vi "TestM1M3SALTelemetry.vi"() -> ()   [LabVIEW 2016]
uses:
  Communicator/M1M3SAL/M1M3SAL.lvclass
  Communicator/DataTypes/M1M3SALSettings.ctl
  UserEvents/UserEvents.lvclass
  DataTypes/General/ShutdownEvent.ctl
  Communicator/M1M3SAL/M1M3SAL.lvclass/M1M3SAL.ctl
  UserEvents/UserEvents.lvclass/UserEvents.ctl
  DataTypes/Topics/TelemetryAirData.ctl
  DataTypes/Topics/Parts/Timestamp.ctl
  DataTypes/Topics/TelemetryIMSData.ctl
  DataTypes/Topics/TelemetryDynamicData.ctl
  DataTypes/Topics/TelemetryElevationData.ctl
  DataTypes/Topics/TelemetryForceActuatorData.ctl
  DataTypes/Topics/TelemetryForceActuatorStatus.ctl
  DataTypes/Topics/TelemetryFPGAData.ctl
  DataTypes/Topics/TelemetryMirrorForceData.ctl
  DataTypes/Topics/TelemetryHardpointData.ctl
  DataTypes/Topics/TelemetryHardpointStatus.ctl
  Communicator/M1M3SupportCommunicator.lvlib
  DataTypes/Topics/M1M3SupportTopics.lvlib
  DataTypes/General/M1M3SupportGeneral.lvlib
panel:
  out "TelemetryMirrorForceData":bool
  in  "TelemetryMirrorForceDataGo":bool
  out "TelemetryHardpointStatus":bool
  out "TelemetryHardpointData":bool
  out "TelemetryFPGAData":bool
  in  "TelemetryHardpointStatus":bool
  in  "TelemetryHardpointData":bool
  in  "TelemetryFPGADataGo":bool
  out "TelemetryForceActuatorStatus":bool
  out "TelemetryForceActuatorData":bool
  out "TelemetryElevationData":bool
  out "TelemetryDynamicData":bool
  in  "TelemetryForceActuatorStatusGo":bool
  in  "TelemetryForceActuatorDataGo":bool
  in  "TelemetryElevationDataGo":bool
  in  "TelemetryDynamicDataGo":bool
  in  "TelemetryIMSDataGo":bool
  out "TelemetryIMSData":bool
  out "Ready?":bool
  in  "TelemetryAirDataGo":bool
  out "TelemetryAirData":bool
  in  "Stop":bool
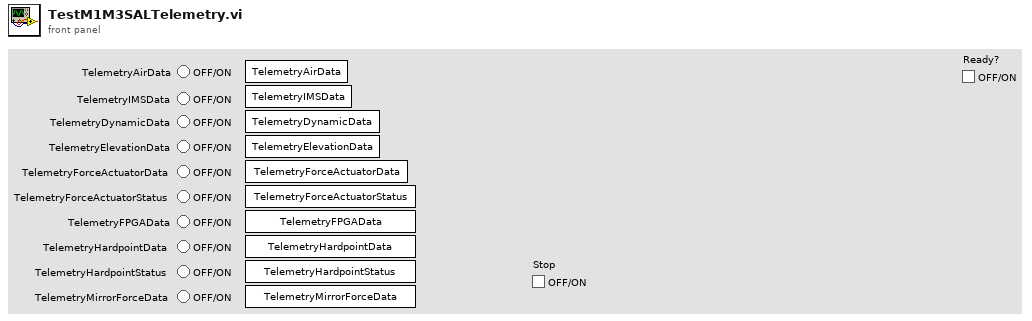
[diagram p1: front panel]
types:
  T1 = typedef "M1M3SupportGeneral.lvlib/ShutdownEvent.ctl" = cluster{"Shutdown":bool}
  T2 = typedef "M1M3SupportCommunicator.lvlib/M1M3SALSettings.ctl" = cluster{"IPAddress":string, "Port":u16, "StartupScript":string}
  T3 = typedef "M1M3SupportTopics.lvlib/Timestamp.ctl" = dbl
  T4 = typedef "M1M3SupportTypes.lvlib/Timestamp.ctl" = dbl
  T5 = typedef "M1M3SupportTopics.lvlib/TelemetryAirData.ctl" = cluster{"Timestamp":T3, "CellAirPressure":sgl, "HardpointAirPressure":sgl}
  T6 = typedef "M1M3SupportTopics.lvlib/TelemetryIMSData.ctl" = cluster{"Timestamp":T3, "XPosition":dbl, "YPosition":dbl, "ZPosition":dbl, "XRotation":dbl, "YRotation":dbl, "ZRotation":dbl}
  T7 = typedef "M1M3SupportTopics.lvlib/TelemetryDynamicData.ctl" = cluster{"Timestamp":T3, "AzimuthVelocity":dbl, "ElevationVelocity":dbl, "AzimuthAcceleration":dbl, "ElevationAcceleration":dbl}
  T8 = typedef "M1M3SupportTopics.lvlib/TelemetryElevationData.ctl" = cluster{"Timestamp":T3, "InclinometerElevation":dbl, "MeasuredElevation":dbl}
  T9 = typedef "M1M3SupportTopics.lvlib/TelemetryForceActuatorData.ctl" = cluster{"Timestamp":T3, "SlewFlagCommanded":bool[], "XSetpointCommanded":dbl[], "YSetpointCommanded":dbl[], "ZSetpointCommanded":dbl[], "XForce":sgl[], "YForce":sgl[], "ZForce":sgl[], "ILCFault":bool[], "DCAFault":bool[], "BroadcastCounter":u8[]}
  T10 = typedef "M1M3SupportTopics.lvlib/TelemetryForceActuatorStatus.ctl" = cluster{"Timestamp":T3, "Mode":u8[], "MajorFault":bool[], "MinorFault":bool[], "FaultOverridden":bool[], "DCAFault":bool[], "WatchdogReset":bool[], "BrownoutDetected":bool[], "EventTrapReset":bool[], "MotorPowerFault":bool[], "SSRPowerFault":bool[], "AUXPowerFault":bool[], "SMCPowerFault":bool[], "DCAOutputsEnabled":bool[], "DCAPowerFault":bool[], "DCAAmplifierAFault":bool[], "DCAAmplifierBFault":bool[], "DCAEventTrapReset":bool[]}
  T11 = typedef "M1M3SupportTopics.lvlib/TelemetryFPGAData.ctl" = cluster{"Timestamp":T3, "ModbusSubnetATxInternalFIFOOverflow":bool, "ModbusSubnetAInvalidInstruction":bool, "ModbusSubnetAWaitForRxFrameTimeout":bool, "ModbusSubnetAStartBitError":bool, "ModbusSubnetAStopBitError":bool, "ModbusSubnetARxDataFIFOOverflow":bool, "ModbusSubnetATxByteCount":u32, "ModbusSubnetATxFrameCount":u32, "ModbusSubnetARxByteCount":u32, "ModbusSubnetARxFrameCount":u32, "ModbusSubnetBTxInternalFIFOOverflow":bool, "ModbusSubnetBInvalidInstruction":bool, "ModbusSubnetBWaitForRxFrameTimeout":bool, "ModbusSubnetBStartBitError":bool, "ModbusSubnetBStopBitError":bool, "ModbusSubnetBRxDataFIFOOverflow":bool, "ModbusSubnetBTxByteCount":u32, "ModbusSubnetBTxFrameCount":u32, "ModbusSubnetBRxByteCount":u32, "ModbusSubnetBRxFrameCount":u32, "ModbusSubnetCTxInternalFIFOOverflow":bool, "ModbusSubnetCInvalidInstruction":bool, "ModbusSubnetCWaitForRxFrameTimeout":bool, "ModbusSubnetCStartBitError":bool, "ModbusSubnetCStopBitError":bool, "ModbusSubnetCRxDataFIFOOverflow":bool, "ModbusSubnetCTxByteCount":u32, "ModbusSubnetCTxFrameCount":u32, "ModbusSubnetCRxByteCount":u32, "ModbusSubnetCRxFrameCount":u32, "ModbusSubnetDTxInternalFIFOOverflow":bool, "ModbusSubnetDInvalidInstruction":bool, "ModbusSubnetDWaitForRxFrameTimeout":bool, "ModbusSubnetDStartBitError":bool, "ModbusSubnetDStopBitError":bool, "ModbusSubnetDRxDataFIFOOverflow":bool, "ModbusSubnetDTxByteCount":u32, "ModbusSubnetDTxFrameCount":u32, "ModbusSubnetDRxByteCount":u32, "ModbusSubnetDRxFrameCount":u32, "ModbusSubnetETxInternalFIFOOverflow":bool, "ModbusSubnetEInvalidInstruction":bool, "ModbusSubnetEWaitForRxFrameTimeout":bool, "ModbusSubnetEStartBitError":bool, "ModbusSubnetEStopBitError":bool, "ModbusSubnetERxDataFIFOOverflow":bool, "ModbusSubnetETxByteCount":u32, "ModbusSubnetETxFrameCount":u32, "ModbusSubnetERxByteCount":u32, "ModbusSubnetERxFrameCount":u32, "FPGATimestamp":dbl}
  T12 = typedef "M1M3SupportTopics.lvlib/TelemetryMirrorForceData.ctl" = cluster{"Timestamp":T3, "Fx":dbl, "Fy":dbl, "Fz":dbl, "Mx":dbl, "My":dbl, "Mz":dbl}
  T13 = typedef "M1M3SupportTopics.lvlib/TelemetryHardpointData.ctl" = cluster{"Timestamp":T3, "StepsCommanded":i16[], "Force":sgl[], "Encoder":i32[], "ILCFault":bool[], "CWLimitOperated":bool[], "CCWLimitOperated":bool[], "BroadcastCounter":u8[]}
  T14 = typedef "M1M3SupportTopics.lvlib/TelemetryHardpointStatus.ctl" = cluster{"Timestamp":T3, "Mode":u8[], "MajorFault":bool[], "MinorFault":bool[], "FaultOverridden":bool[], "WatchdogReset":bool[], "BrownoutDetected":bool[], "EventTrapReset":bool[], "MotorPowerFault":bool[], "SSRPowerFault":bool[], "AUXPowerFault":bool[], "SMCPowerFault":bool[]}
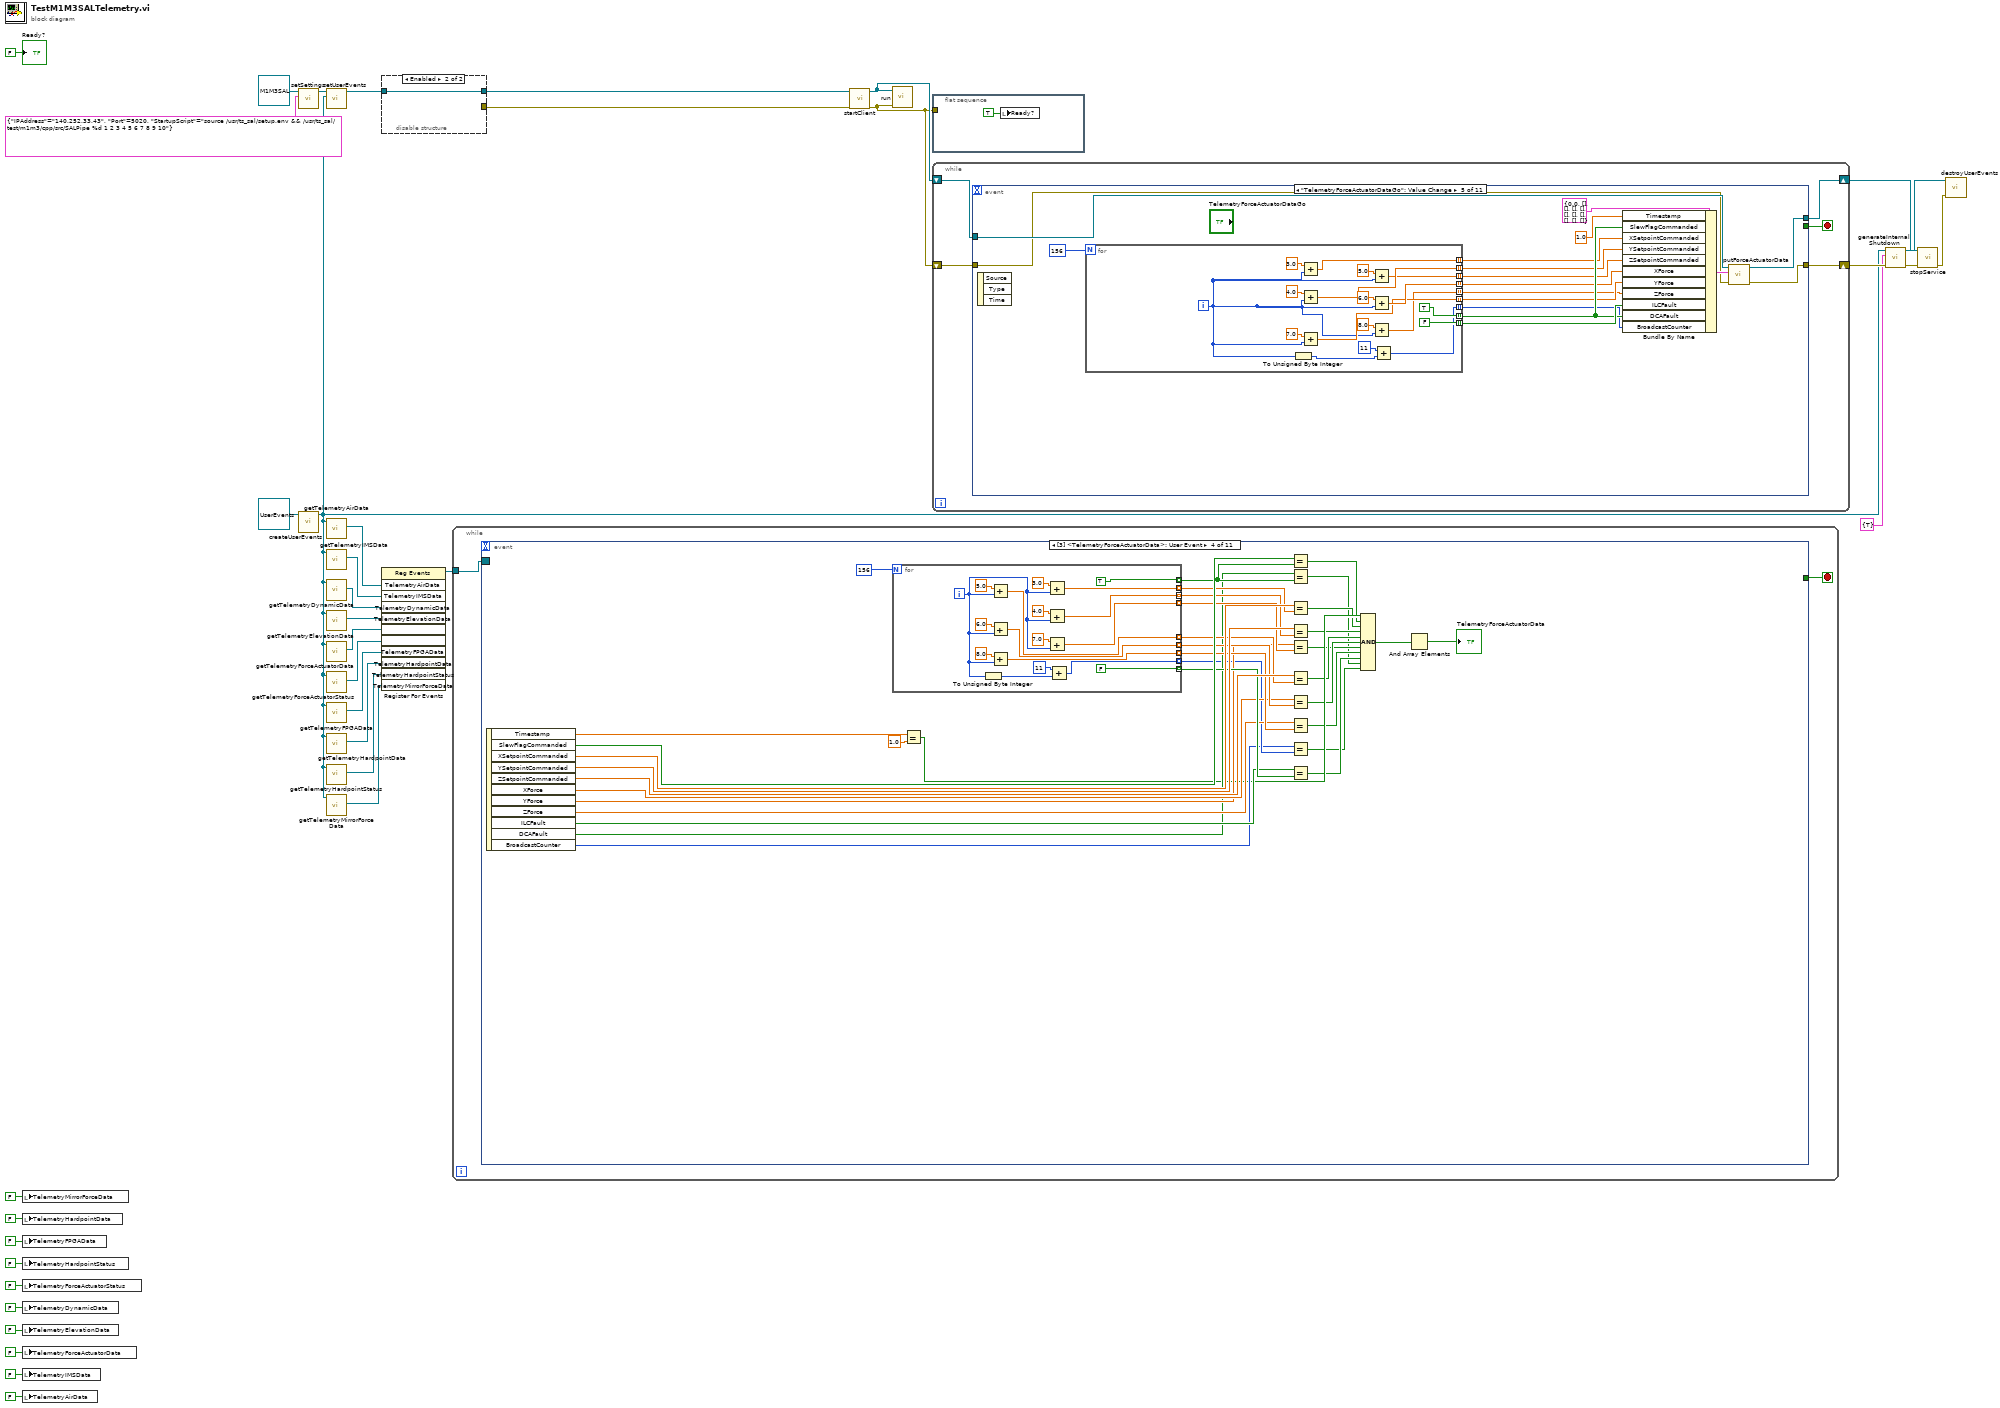
[diagram p0: block diagram]
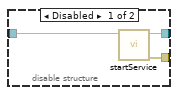
[diagram p2: hidden frame]
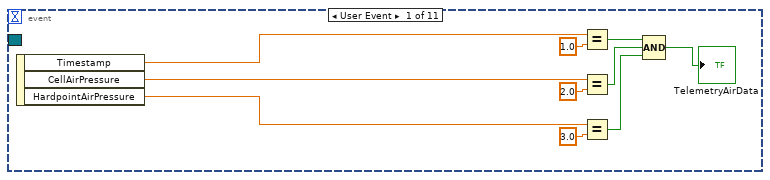
[diagram p3: hidden frame]
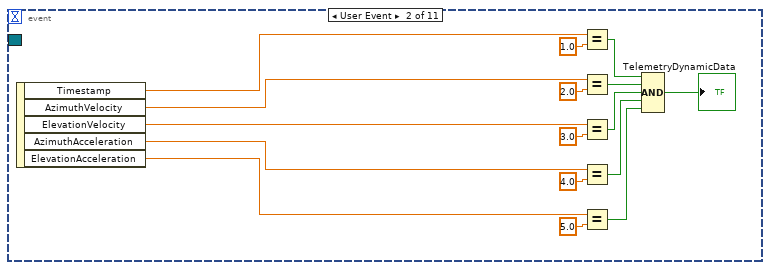
[diagram p4: hidden frame]
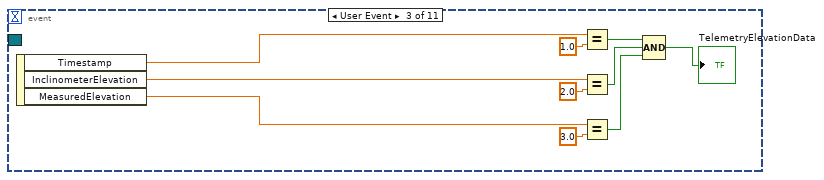
[diagram p5: hidden frame]
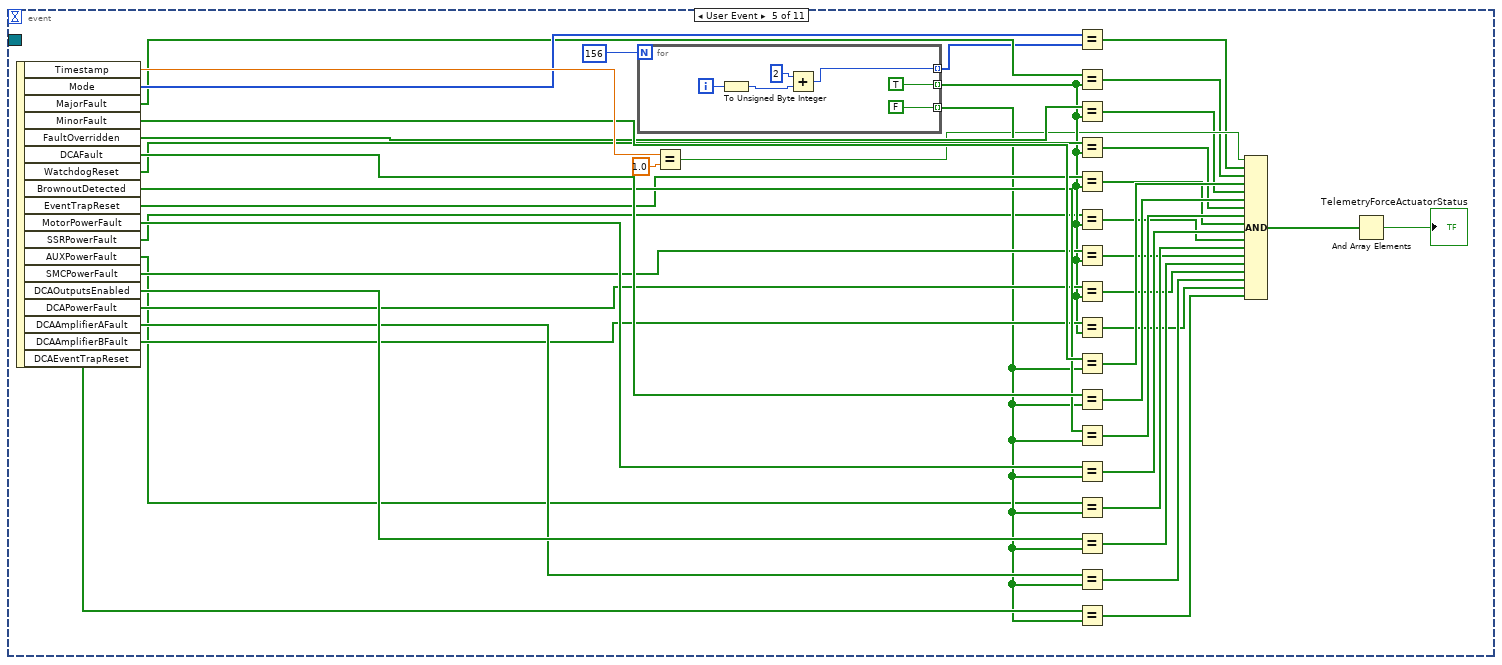
[diagram p6: hidden frame]
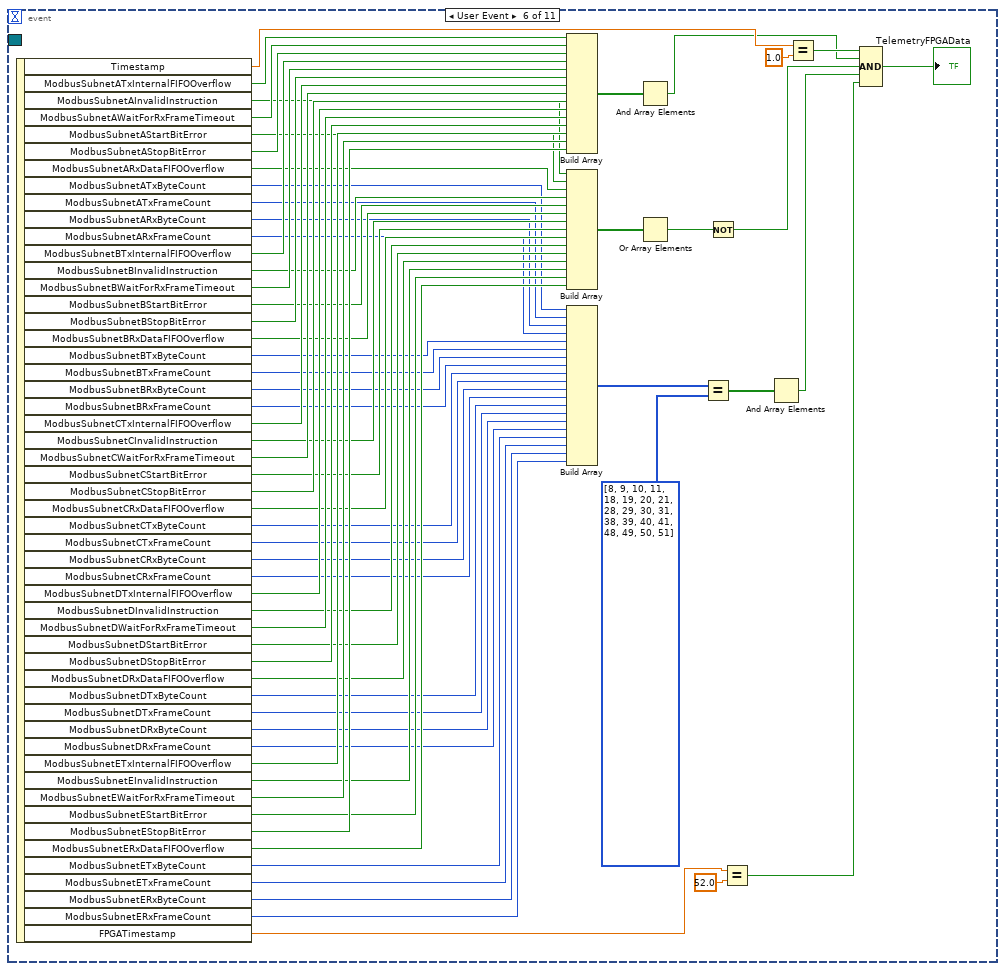
[diagram p7: hidden frame]
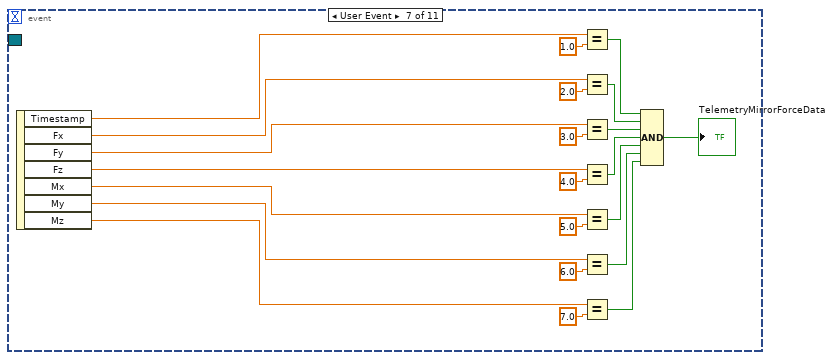
[diagram p8: hidden frame]
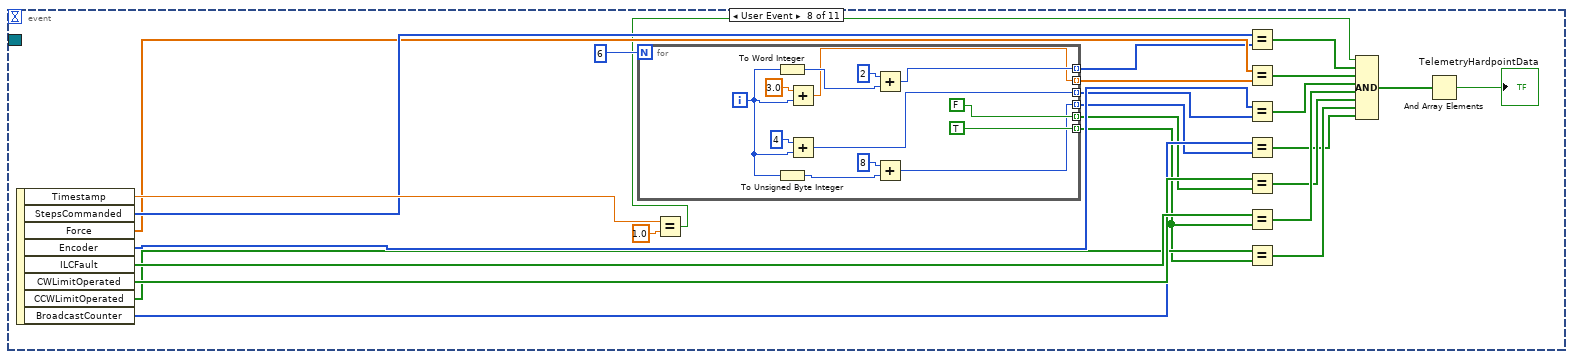
[diagram p9: hidden frame]
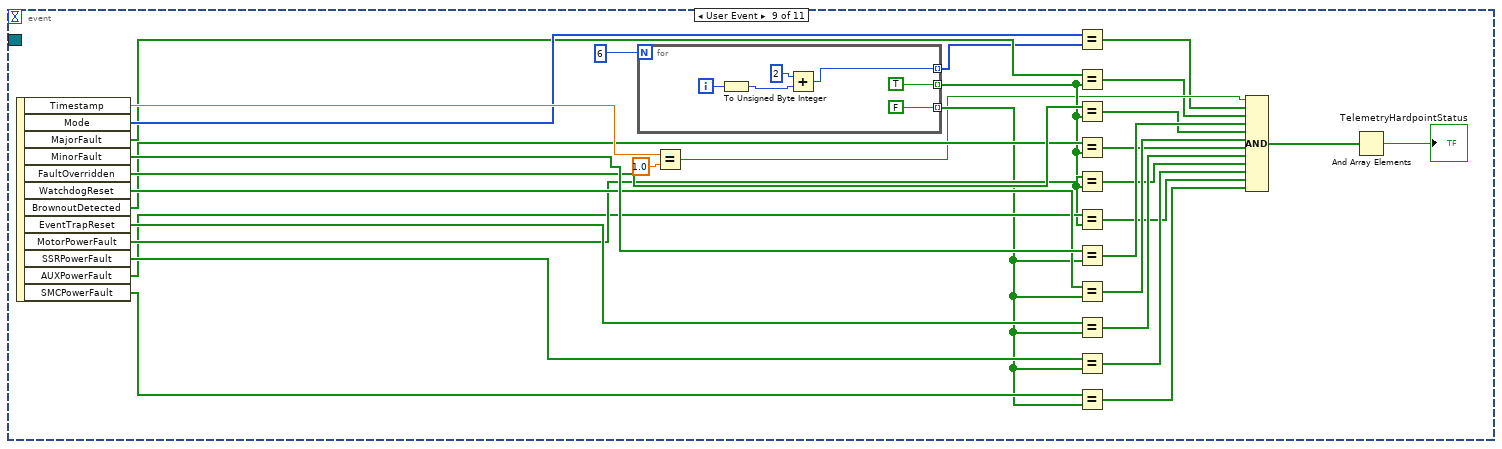
[diagram p10: hidden frame]
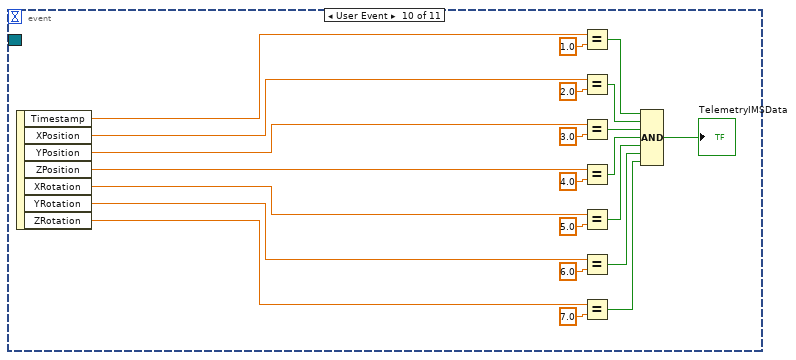
[diagram p11: hidden frame]
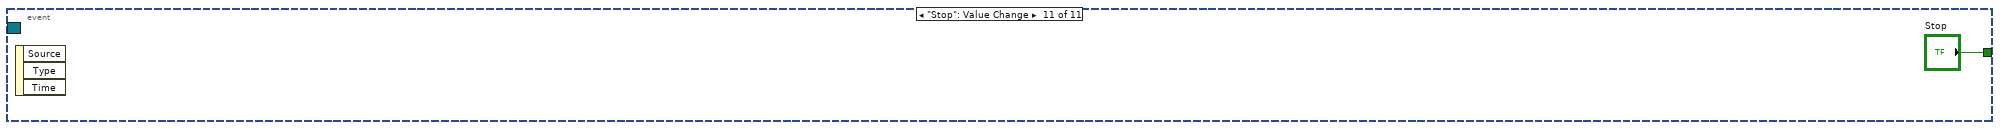
[diagram p12: hidden frame]
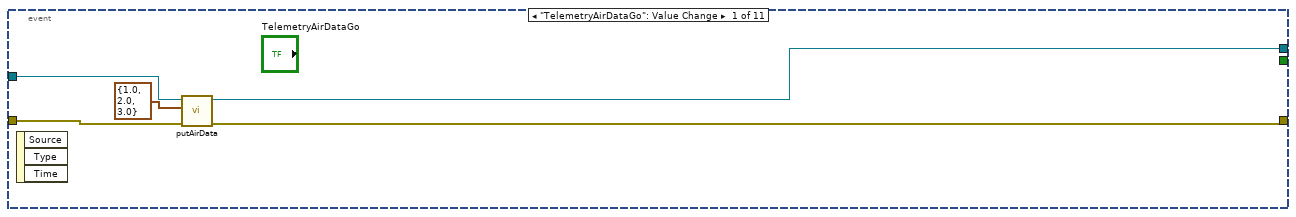
[diagram p13: hidden frame]
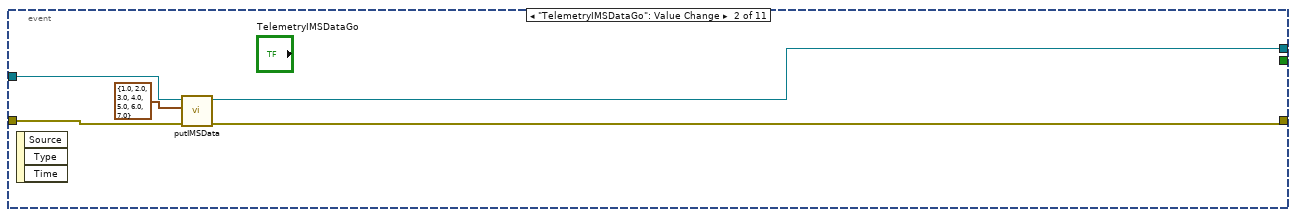
[diagram p14: hidden frame]
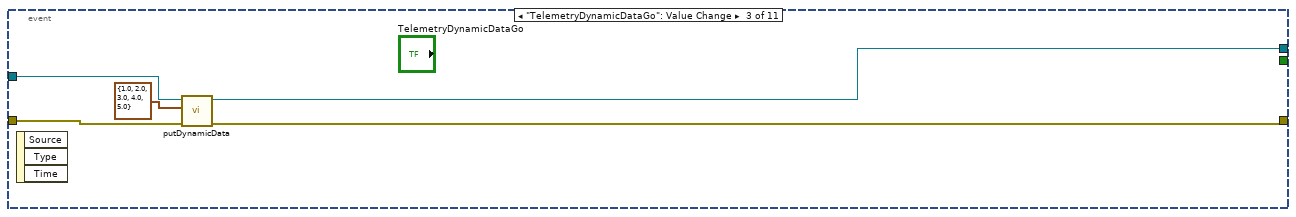
[diagram p15: hidden frame]
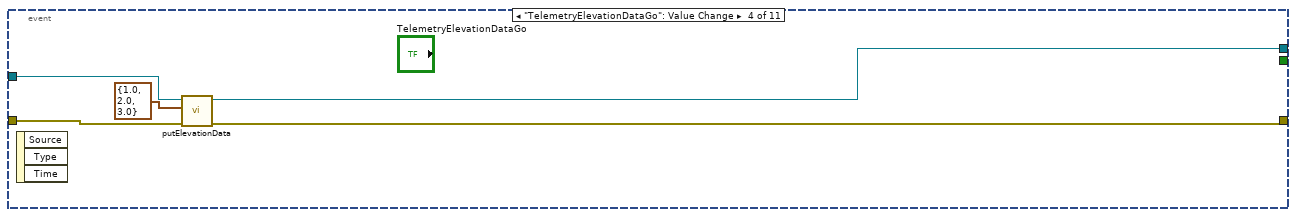
[diagram p16: hidden frame]
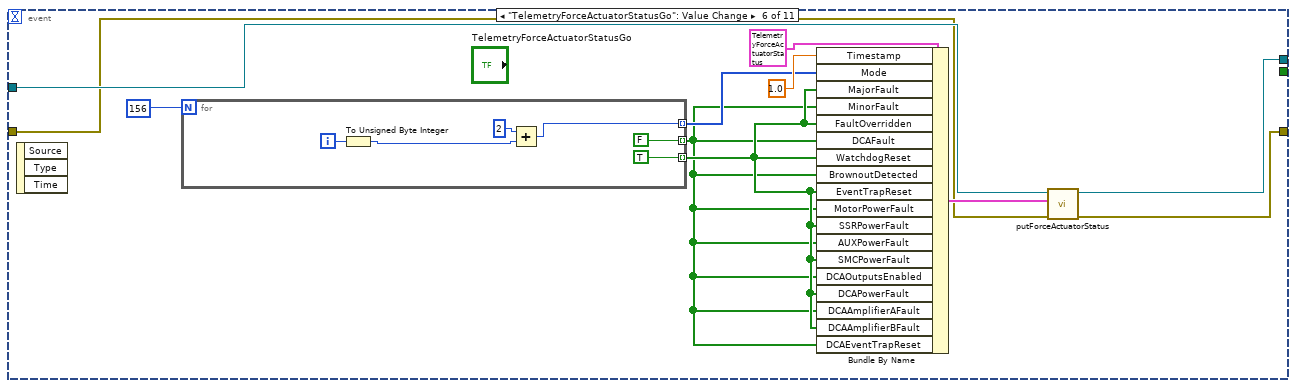
[diagram p17: hidden frame]
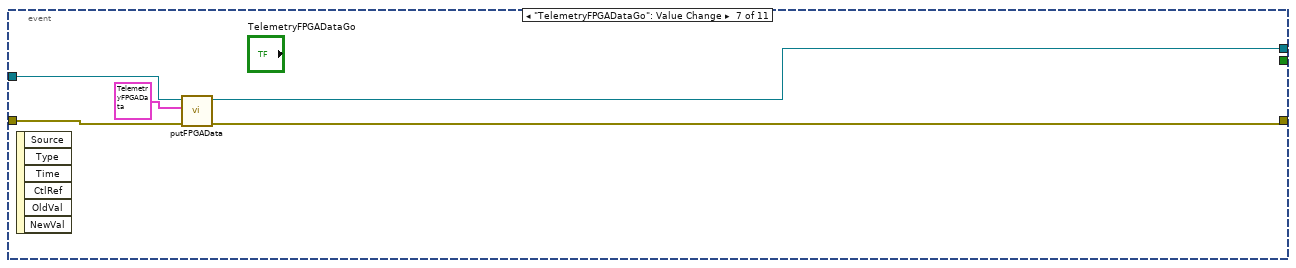
[diagram p18: hidden frame]
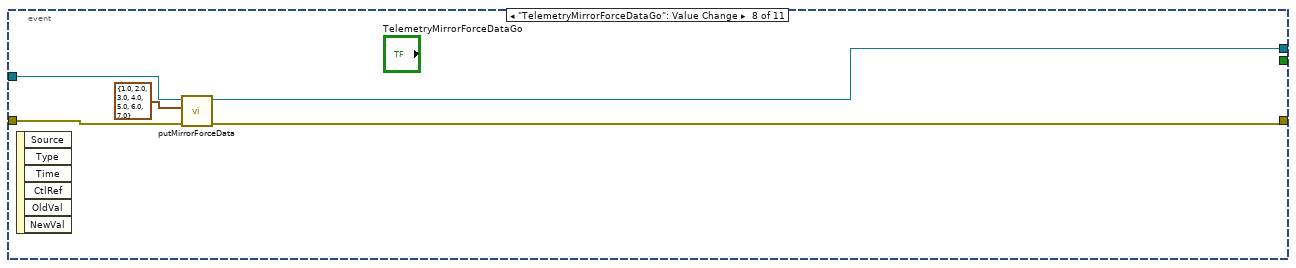
[diagram p19: hidden frame]
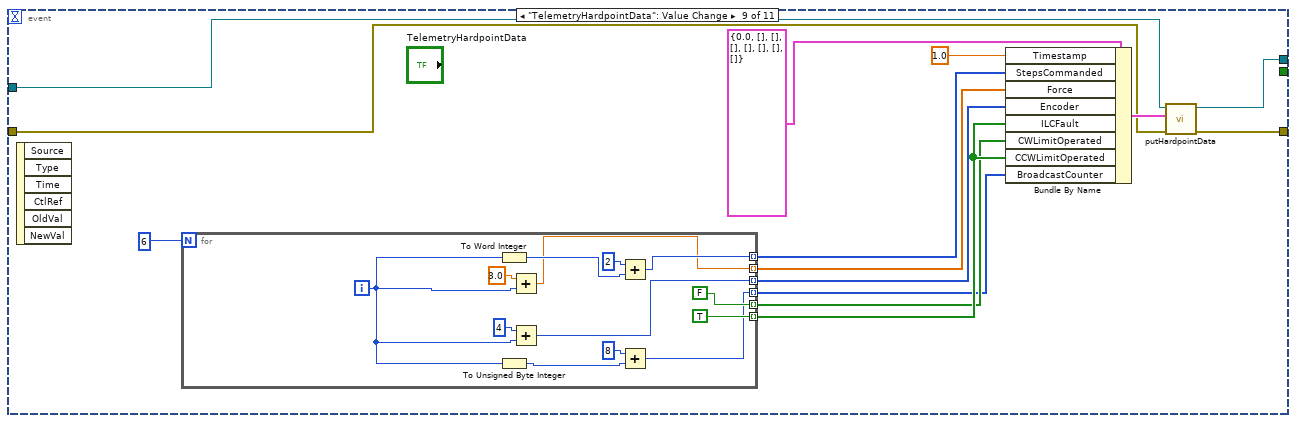
[diagram p20: hidden frame]
diagram:
  n1 = local write "TelemetryMirrorForceData"(FALSE ("TelemetryMirrorForceData")) -> ()
  n2 = local write "TelemetryHardpointData"(FALSE ("TelemetryHardpointData")) -> ()
  n3 = local write "TelemetryFPGAData"(FALSE ("TelemetryFPGAData")) -> ()
  n4 = local write "TelemetryHardpointStatus"(FALSE ("TelemetryHardpointStatus")) -> ()
  n5 = local write "TelemetryForceActuatorStatus"(FALSE ("TelemetryForceActuatorStatus")) -> ()
  n6 = local write "TelemetryDynamicData"(FALSE ("TelemetryDynamicData")) -> ()
  n7 = local write "TelemetryElevationData"(FALSE ("TelemetryElevationData")) -> ()
  n8 = local write "TelemetryForceActuatorData"(FALSE ("TelemetryForceActuatorData")) -> ()
  n9 = local write "TelemetryIMSData"(FALSE ("TelemetryIMSData")) -> ()
  n10 = local write "TelemetryAirData"(FALSE ("TelemetryAirData")) -> ()
  n11 = call "setSettings.vi"("Settings"=T2 {"IPAddress"="140.252.33.43", "Port"=5020, "StartupScript"="source /usr/ts_sal/setup.env && /usr/ts_sal/test/m1m3/cpp/src/SALPipe %d 1 2 3 4 5 6 7 8 9 10"}, "M1M3SAL in"=refnum<class "M1M3SAL.lvclass"> refnum ("M1M3SupportCommunicator.lvlib:M1M3SAL.lvclass")) -> ("M1M3SAL out"=w35:refnum<class "M1M3SAL.lvclass">)  [unwired: 9 in]
  n12 = call "createUserEvents.vi"("UserEvents in"=refnum<class "UserEvents.lvclass"> refnum ("UserEvents.lvclass")) -> ("UserEvents out"=w22:refnum<class "UserEvents.lvclass">)  [unwired: 9 in, 1 out]
  n13 = call "setUserEvents.vi"("UserEvents"=w22, "M1M3SAL in"=w35) -> ("M1M3SAL out"=w34:refnum<class "M1M3SAL.lvclass">)  [unwired: 9 in]
  n14 = call "getTelemetryAirData.vi"("UserEvents in"=w22) -> ("TelemetryAirData"=w32:refnum<user-event>)  [unwired: 9 in, 1 out]
  n15 = call "getTelemetryIMSData.vi"("UserEvents in"=w22) -> ("TelemetryIMSData"=w21:refnum<user-event>)  [unwired: 9 in, 1 out]
  n16 = call "getTelemetryDynamicData.vi"("UserEvents in"=w22) -> ("TelemetryDynamicData"=w20:refnum<user-event>)  [unwired: 9 in, 1 out]
  n17 = call "getTelemetryElevationData.vi"("UserEvents in"=w22) -> ("TelemetryElevationData"=w19:refnum<user-event>)  [unwired: 9 in, 1 out]
  n18 = call "getTelemetryForceActuatorData.vi"("UserEvents in"=w22) -> ("TelemetryForceActuatorData"=w18:refnum<user-event>)  [unwired: 9 in, 1 out]
  n19 = call "getTelemetryForceActuatorStatus.vi"("UserEvents in"=w22) -> ("TelemetryForceActuatorStatus"=w17:refnum<user-event>)  [unwired: 9 in, 1 out]
  n20 = call "getTelemetryFPGAData.vi"("UserEvents in"=w22) -> ("TelemetryFPGAData"=w16:refnum<user-event>)  [unwired: 9 in, 1 out]
  n21 = call "getTelemetryHardpointData.vi"("UserEvents in"=w22) -> ("TelemetryHardpointData"=w15:refnum<user-event>)  [unwired: 9 in, 1 out]
  n22 = call "getTelemetryHardpointStatus.vi"("UserEvents in"=w22) -> ("TelemetryHardpointStatus"=w14:refnum<user-event>)  [unwired: 9 in, 1 out]
  n23 = call "getTelemetryMirrorForceData.vi"("UserEvents in"=w22) -> ("TelemetryMirrorForceData"=w13:refnum<user-event>)  [unwired: 9 in, 1 out]
  n24 = disable-structure shown="Enabled" {
    disable-tunnel: w34 -> [w41 w42]
    disable-tunnel: [w40 w42] -> w33
    disable-tunnel: [w39 _] -> w30
    frame Disabled {
      n25 = call-dynamic "startService.vi"("M1M3SAL in"=w41) -> ("error out"=w39:errorcluster, "M1M3SAL out"=w40:refnum<class "M1M3SAL.lvclass">)  [unwired: 9 in]
    }
    frame Enabled {
    }
  }
  n26 = register-events(w32, w21, w20, w19, w18, w17, w16, w15, w14, w13) -> (reference out=w31:refnum<event-registration>)  [unwired: 2 in, 1 out]
  n27 = while {
    tunnel: w31 -> [w44]
    stop <- w43 stop-if-true
    n28 = event shown="[3] <TelemetryForceActuatorData>: User Event" {
      selector: w44 -> [_ _ _ _ _ _ _ _ _ _ _]
      dyn-events: _ -> [_ _ _ _ _ _ _ _ _ _ _]
      timeout: _ -> [_ _ _ _ _ _ _ _ _ _ _]
      tunnel: [_ _ _ _ _ _ _ _ _ _ "Stop"] -> w43
      event User Event {
        n29 = event-data() -> ("Timestamp"=w54:T3, "CellAirPressure"=w53:sgl, "HardpointAirPressure"=w52:sgl)  [unwired: 1 in]
        n30 = Equal?(x=w54, y=T3 1.0) -> (x = y?=w48:bool)
        n31 = Equal?(x=w53, y=sgl 2.0) -> (x = y?=w47:bool)
        n32 = Equal?(x=w52, y=sgl 3.0) -> (x = y?=w46:bool)
        n33 = Compound Arithmetic op=AND(w48, w47, w46) -> (→"TelemetryAirData":bool)
      }
      event User Event {
        n34 = event-data() -> ("Timestamp"=w70:T3, "AzimuthVelocity"=w69:dbl, "ElevationVelocity"=w68:dbl, "AzimuthAcceleration"=w67:dbl, "ElevationAcceleration"=w66:dbl)  [unwired: 1 in]
        n35 = Equal?(x=w70, y=T3 1.0) -> (x = y?=w60:bool)
        n36 = Equal?(x=w69, y=2.0) -> (x = y?=w59:bool)
        n37 = Equal?(x=w68, y=3.0) -> (x = y?=w58:bool)
        n38 = Equal?(x=w67, y=4.0) -> (x = y?=w57:bool)
        n39 = Equal?(x=w66, y=5.0) -> (x = y?=w56:bool)
        n40 = Compound Arithmetic op=AND(w60, w59, w58, w57, w56) -> (→"TelemetryDynamicData":bool)
      }
      event User Event {
        n41 = event-data() -> ("Timestamp"=w80:T3, "InclinometerElevation"=w79:dbl, "MeasuredElevation"=w78:dbl)  [unwired: 1 in]
        n42 = Equal?(x=w80, y=T3 1.0) -> (x = y?=w74:bool)
        n43 = Equal?(x=w79, y=2.0) -> (x = y?=w73:bool)
        n44 = Equal?(x=w78, y=3.0) -> (x = y?=w72:bool)
        n45 = Compound Arithmetic op=AND(w74, w73, w72) -> (→"TelemetryElevationData":bool)
      }
      event User Event {
        n46 = event-data() -> ("Timestamp"=w114:T3, "SlewFlagCommanded"=w112:bool[], "XSetpointCommanded"=w111:dbl[], "YSetpointCommanded"=w109:dbl[], "ZSetpointCommanded"=w107:dbl[], "XForce"=w101:sgl[], "YForce"=w100:sgl[], "ZForce"=w99:sgl[], "ILCFault"=w98:bool[], "DCAFault"=w96:bool[], "BroadcastCounter"=w94:u8[])  [unwired: 1 in]
        n47 = for {
          N: 156 -> [_]
          tunnel: [TRUE] -> w97 mode=indexing
          tunnel: [FALSE] -> w102 mode=indexing
          tunnel: [w130] -> w110 mode=indexing
          tunnel: [w128] -> w108 mode=indexing
          tunnel: [w123] -> w106 mode=indexing
          tunnel: [w122] -> w105 mode=indexing
          tunnel: [w121] -> w104 mode=indexing
          tunnel: [w120] -> w103 mode=indexing
          tunnel: [w116] -> w95 mode=indexing
          i -> [w119]
          n48 = To Unsigned Byte Integer(number=w119) -> (unsigned 8bit integer=w118:u8)
          n49 = Add(x=5.0, y=w119) -> (x+y=w123:dbl)
          n50 = Add(x=sgl 6.0, y=w119) -> (x+y=w122:sgl)
          n51 = Add(x=sgl 8.0, y=w119) -> (x+y=w120:sgl)
          n52 = Add(x=3.0, y=w119) -> (x+y=w130:dbl)
          n53 = Add(x=4.0, y=w119) -> (x+y=w128:dbl)
          n54 = Add(x=sgl 7.0, y=w119) -> (x+y=w121:sgl)
          n55 = Add(x=u8 11, y=w118) -> (x+y=w116:u8)
        }
        n56 = Equal?(x=w114, y=T3 1.0) -> (x = y?=w93:bool)
        n57 = Equal?(x=w112, y=w97) -> (x = y?=w92:bool[])
        n58 = Equal?(x=w96, y=w97) -> (x = y?=w84:bool[])
        n59 = Equal?(x=w111, y=w110) -> (x = y?=w91:bool[])
        n60 = Equal?(x=w109, y=w108) -> (x = y?=w90:bool[])
        n61 = Equal?(x=w100, y=w104) -> (x = y?=w87:bool[])
        n62 = Equal?(x=w107, y=w106) -> (x = y?=w89:bool[])
        n63 = Equal?(x=w101, y=w105) -> (x = y?=w88:bool[])
        n64 = Equal?(x=w99, y=w103) -> (x = y?=w86:bool[])
        n65 = Equal?(x=w94, y=w95) -> (x = y?=w83:bool[])
        n66 = Equal?(x=w98, y=w102) -> (x = y?=w85:bool[])
        n67 = Compound Arithmetic op=AND(w93, w92, w91, w90, w89, w88, w87, w86, w85, w84, w83) -> (w82:bool[])
        n68 = And Array Elements(Boolean array=w82) -> (logical AND=→"TelemetryForceActuatorData":bool)
      }
      event User Event {
        n69 = event-data() -> ("Timestamp"=w175:T3, "Mode"=w174:u8[], "MajorFault"=w173:bool[], "MinorFault"=w172:bool[], "FaultOverridden"=w171:bool[], "DCAFault"=w170:bool[], "WatchdogReset"=w169:bool[], "BrownoutDetected"=w168:bool[], "EventTrapReset"=w167:bool[], "MotorPowerFault"=w166:bool[], "SSRPowerFault"=w134:bool[], "AUXPowerFault"=w135:bool[], "SMCPowerFault"=w165:bool[], "DCAOutputsEnabled"=w164:bool[], "DCAPowerFault"=w163:bool[], "DCAAmplifierAFault"=w162:bool[], "DCAAmplifierBFault"=w161:bool[], "DCAEventTrapReset"=w160:bool[])  [unwired: 1 in]
        n70 = for {
          N: 156 -> [_]
          tunnel: [w179] -> w159 mode=indexing
          tunnel: [TRUE] -> w158 mode=indexing
          tunnel: [FALSE] -> w157 mode=indexing
          i -> [w182]
          n71 = To Unsigned Byte Integer(number=w182) -> (unsigned 8bit integer=w181:u8)
          n72 = Add(x=u8 2, y=w181) -> (x+y=w179:u8)
        }
        n73 = Equal?(x=w175, y=T3 1.0) -> (x = y?=w155:bool)
        n74 = Equal?(x=w174, y=w159) -> (x = y?=w154:bool[])
        n75 = Equal?(x=w173, y=w158) -> (x = y?=w153:bool[])
        n76 = Equal?(x=w171, y=w158) -> (x = y?=w151:bool[])
        n77 = Equal?(x=w169, y=w158) -> (x = y?=w149:bool[])
        n78 = Equal?(x=w167, y=w158) -> (x = y?=w147:bool[])
        n79 = Equal?(x=w134, y=w158) -> (x = y?=w145:bool[])
        n80 = Equal?(x=w165, y=w158) -> (x = y?=w143:bool[])
        n81 = Equal?(x=w163, y=w158) -> (x = y?=w141:bool[])
        n82 = Equal?(x=w161, y=w158) -> (x = y?=w139:bool[])
        n83 = Equal?(x=w172, y=w157) -> (x = y?=w152:bool[])
        n84 = Equal?(x=w170, y=w157) -> (x = y?=w150:bool[])
        n85 = Equal?(x=w168, y=w157) -> (x = y?=w148:bool[])
        n86 = Equal?(x=w166, y=w157) -> (x = y?=w146:bool[])
        n87 = Equal?(x=w135, y=w157) -> (x = y?=w144:bool[])
        n88 = Equal?(x=w164, y=w157) -> (x = y?=w142:bool[])
        n89 = Equal?(x=w162, y=w157) -> (x = y?=w140:bool[])
        n90 = Equal?(x=w160, y=w157) -> (x = y?=w138:bool[])
        n91 = Compound Arithmetic op=AND(w155, w154, w153, w152, w151, w150, w149, w148, w147, w146, w145, w144, w143, w142, w141, w140, w139, w138) -> (w137:bool[])
        n92 = And Array Elements(Boolean array=w137) -> (logical AND=→"TelemetryForceActuatorStatus":bool)
      }
      event User Event {
        n93 = event-data() -> ("Timestamp"=w216:T3, "ModbusSubnetATxInternalFIFOOverflow"=w248:bool, "ModbusSubnetAInvalidInstruction"=w232:bool, "ModbusSubnetAWaitForRxFrameTimeout"=w247:bool, "ModbusSubnetAStartBitError"=w230:bool, "ModbusSubnetAStopBitError"=w246:bool, "ModbusSubnetARxDataFIFOOverflow"=w229:bool, "ModbusSubnetATxByteCount"=w214:u32, "ModbusSubnetATxFrameCount"=w213:u32, "ModbusSubnetARxByteCount"=w212:u32, "ModbusSubnetARxFrameCount"=w211:u32, "ModbusSubnetBTxInternalFIFOOverflow"=w245:bool, "ModbusSubnetBInvalidInstruction"=w228:bool, "ModbusSubnetBWaitForRxFrameTimeout"=w244:bool, "ModbusSubnetBStartBitError"=w227:bool, "ModbusSubnetBStopBitError"=w243:bool, "ModbusSubnetBRxDataFIFOOverflow"=w226:bool, "ModbusSubnetBTxByteCount"=w210:u32, "ModbusSubnetBTxFrameCount"=w209:u32, "ModbusSubnetBRxByteCount"=w208:u32, "ModbusSubnetBRxFrameCount"=w207:u32, "ModbusSubnetCTxInternalFIFOOverflow"=w242:bool, "ModbusSubnetCInvalidInstruction"=w225:bool, "ModbusSubnetCWaitForRxFrameTimeout"=w241:bool, "ModbusSubnetCStartBitError"=w224:bool, "ModbusSubnetCStopBitError"=w240:bool, "ModbusSubnetCRxDataFIFOOverflow"=w223:bool, "ModbusSubnetCTxByteCount"=w206:u32, "ModbusSubnetCTxFrameCount"=w205:u32, "ModbusSubnetCRxByteCount"=w204:u32, "ModbusSubnetCRxFrameCount"=w203:u32, "ModbusSubnetDTxInternalFIFOOverflow"=w239:bool, "ModbusSubnetDInvalidInstruction"=w222:bool, "ModbusSubnetDWaitForRxFrameTimeout"=w238:bool, "ModbusSubnetDStartBitError"=w221:bool, "ModbusSubnetDStopBitError"=w237:bool, "ModbusSubnetDRxDataFIFOOverflow"=w220:bool, "ModbusSubnetDTxByteCount"=w202:u32, "ModbusSubnetDTxFrameCount"=w201:u32, "ModbusSubnetDRxByteCount"=w200:u32, "ModbusSubnetDRxFrameCount"=w199:u32, "ModbusSubnetETxInternalFIFOOverflow"=w236:bool, "ModbusSubnetEInvalidInstruction"=w219:bool, "ModbusSubnetEWaitForRxFrameTimeout"=w235:bool, "ModbusSubnetEStartBitError"=w218:bool, "ModbusSubnetEStopBitError"=w234:bool, "ModbusSubnetERxDataFIFOOverflow"=w217:bool, "ModbusSubnetETxByteCount"=w198:u32, "ModbusSubnetETxFrameCount"=w197:u32, "ModbusSubnetERxByteCount"=w196:u32, "ModbusSubnetERxFrameCount"=w195:u32, "FPGATimestamp"=w190:dbl)  [unwired: 1 in]
        n94 = Build Array(w248, w247, w246, w245, w244, w243, w242, w241, w240, w239, w238, w237, w236, w235, w234) -> (w233:bool[])
        n95 = Build Array(w232, w230, w229, w228, w227, w226, w225, w224, w223, w222, w221, w220, w219, w218, w217) -> (w231:bool[])
        n96 = Build Array(w214, w213, w212, w211, w210, w209, w208, w207, w206, w205, w204, w203, w202, w201, w200, w199, w198, w197, w196, w195) -> (w192:u32[])
        n97 = And Array Elements(Boolean array=w233) -> (logical AND=w187:bool)
        n98 = Or Array Elements(Boolean array=w231) -> (logical OR=w194:bool)
        n99 = Equal?(x=w192, y=u32[] [8, 9, 10, 11, 18, 19, 20, 21, 28, 29, 30, 31, 38, 39, 40, 41, 48, 49, 50, 51]) -> (x = y?=w191:bool[])
        n100 = Not(x=w194) -> (.not. x?=w186:bool)
        n101 = Equal?(x=w190, y=52.0) -> (x = y?=w184:bool)
        n102 = And Array Elements(Boolean array=w191) -> (logical AND=w185:bool)
        n103 = Equal?(x=w216, y=T3 1.0) -> (x = y?=w188:bool)
        n104 = Compound Arithmetic op=AND(w188, w187, w186, w185, w184) -> (→"TelemetryFPGAData":bool)
      }
      event User Event {
        n105 = event-data() -> ("Timestamp"=w270:T3, "Fx"=w269:dbl, "Fy"=w268:dbl, "Fz"=w267:dbl, "Mx"=w266:dbl, "My"=w265:dbl, "Mz"=w264:dbl)  [unwired: 1 in]
        n106 = Equal?(x=w270, y=T3 1.0) -> (x = y?=w256:bool)
        n107 = Equal?(x=w269, y=2.0) -> (x = y?=w255:bool)
        n108 = Equal?(x=w268, y=3.0) -> (x = y?=w254:bool)
        n109 = Equal?(x=w267, y=4.0) -> (x = y?=w253:bool)
        n110 = Equal?(x=w266, y=5.0) -> (x = y?=w252:bool)
        n111 = Equal?(x=w265, y=6.0) -> (x = y?=w251:bool)
        n112 = Equal?(x=w264, y=7.0) -> (x = y?=w250:bool)
        n113 = Compound Arithmetic op=AND(w256, w255, w254, w253, w252, w251, w250) -> (→"TelemetryMirrorForceData":bool)
      }
      event User Event {
        n114 = event-data() -> ("Timestamp"=w295:T4, "StepsCommanded"=w294:i16[], "Force"=w293:sgl[], "Encoder"=w292:i32[], "ILCFault"=w291:bool[], "CWLimitOperated"=w290:bool[], "CCWLimitOperated"=w289:bool[], "BroadcastCounter"=w288:u8[])  [unwired: 1 in]
        n115 = for {
          N: 6 -> [_]
          tunnel: [w307] -> w287 mode=indexing
          tunnel: [w305] -> w286 mode=indexing
          tunnel: [w303] -> w285 mode=indexing
          tunnel: [TRUE] -> w284 mode=indexing
          tunnel: [FALSE] -> w283 mode=indexing
          tunnel: [w297] -> w282 mode=indexing
          i -> [w300]
          n116 = To Word Integer(number=w300) -> (16bit integer=w309:i16)
          n117 = To Unsigned Byte Integer(number=w300) -> (unsigned 8bit integer=w299:u8)
          n118 = Add(x=sgl 3.0, y=w300) -> (x+y=w305:sgl)
          n119 = Add(x=4, y=w300) -> (x+y=w303:i32)
          n120 = Add(x=i16 2, y=w309) -> (x+y=w307:i16)
          n121 = Add(x=u8 8, y=w299) -> (x+y=w297:u8)
        }
        n122 = Equal?(x=w295, y=T3 1.0) -> (x = y?=w281:bool)
        n123 = Equal?(x=w294, y=w287) -> (x = y?=w280:bool[])
        n124 = Equal?(x=w293, y=w286) -> (x = y?=w279:bool[])
        n125 = Equal?(x=w292, y=w285) -> (x = y?=w278:bool[])
        n126 = Equal?(x=w288, y=w282) -> (x = y?=w274:bool[])
        n127 = Equal?(x=w290, y=w283) -> (x = y?=w276:bool[])
        n128 = Equal?(x=w291, y=w284) -> (x = y?=w277:bool[])
        n129 = Equal?(x=w289, y=w284) -> (x = y?=w275:bool[])
        n130 = Compound Arithmetic op=AND(w281, w280, w279, w278, w277, w276, w275, w274) -> (w273:bool[])
        n131 = And Array Elements(Boolean array=w273) -> (logical AND=→"TelemetryHardpointData":bool)
      }
      event User Event {
        n132 = event-data() -> ("Timestamp"=w339:T3, "Mode"=w337:u8[], "MajorFault"=w336:bool[], "MinorFault"=w335:bool[], "FaultOverridden"=w334:bool[], "WatchdogReset"=w333:bool[], "BrownoutDetected"=w332:bool[], "EventTrapReset"=w331:bool[], "MotorPowerFault"=w330:bool[], "SSRPowerFault"=w329:bool[], "AUXPowerFault"=w328:bool[], "SMCPowerFault"=w327:bool[])  [unwired: 1 in]
        n133 = for {
          N: 6 -> [_]
          tunnel: [w343] -> w326 mode=indexing
          tunnel: [FALSE] -> w324 mode=indexing
          tunnel: [TRUE] -> w325 mode=indexing
          i -> [w346]
          n134 = To Unsigned Byte Integer(number=w346) -> (unsigned 8bit integer=w345:u8)
          n135 = Add(x=u8 2, y=w345) -> (x+y=w343:u8)
        }
        n136 = Equal?(x=w339, y=T3 1.0) -> (x = y?=w323:bool)
        n137 = Equal?(x=w337, y=w326) -> (x = y?=w322:bool[])
        n138 = Equal?(x=w336, y=w325) -> (x = y?=w321:bool[])
        n139 = Equal?(x=w334, y=w325) -> (x = y?=w319:bool[])
        n140 = Equal?(x=w332, y=w325) -> (x = y?=w317:bool[])
        n141 = Equal?(x=w330, y=w325) -> (x = y?=w315:bool[])
        n142 = Equal?(x=w328, y=w325) -> (x = y?=w313:bool[])
        n143 = Equal?(x=w335, y=w324) -> (x = y?=w320:bool[])
        n144 = Equal?(x=w333, y=w324) -> (x = y?=w318:bool[])
        n145 = Equal?(x=w331, y=w324) -> (x = y?=w316:bool[])
        n146 = Equal?(x=w329, y=w324) -> (x = y?=w314:bool[])
        n147 = Equal?(x=w327, y=w324) -> (x = y?=w312:bool[])
        n148 = Compound Arithmetic op=AND(w323, w322, w321, w320, w319, w318, w317, w316, w315, w314, w313, w312) -> (w311:bool[])
        n149 = And Array Elements(Boolean array=w311) -> (logical AND=→"TelemetryHardpointStatus":bool)
      }
      event User Event {
        n150 = event-data() -> ("Timestamp"=w368:T3, "XPosition"=w367:dbl, "YPosition"=w366:dbl, "ZPosition"=w365:dbl, "XRotation"=w364:dbl, "YRotation"=w363:dbl, "ZRotation"=w362:dbl)  [unwired: 1 in]
        n151 = Equal?(x=w368, y=T3 1.0) -> (x = y?=w354:bool)
        n152 = Equal?(x=w367, y=2.0) -> (x = y?=w353:bool)
        n153 = Equal?(x=w366, y=3.0) -> (x = y?=w352:bool)
        n154 = Equal?(x=w365, y=4.0) -> (x = y?=w351:bool)
        n155 = Equal?(x=w364, y=5.0) -> (x = y?=w350:bool)
        n156 = Equal?(x=w363, y=6.0) -> (x = y?=w349:bool)
        n157 = Equal?(x=w362, y=7.0) -> (x = y?=w348:bool)
        n158 = Compound Arithmetic op=AND(w354, w353, w352, w351, w350, w349, w348) -> (→"TelemetryIMSData":bool)
      }
      event "Stop": Value Change {
        n159 = event-data() -> ()  [unwired: 1 in, 3 out]
      }
    }
  }
  n160 = call-dynamic "startClient.vi"("error in (no error)"=w30, "M1M3SAL in"=w33) -> ("error out"=w11:errorcluster, "M1M3SAL out"=w27:refnum<class "M1M3SAL.lvclass">)  [unwired: 8 in]
  n161 = call-dynamic "run.vi"("error in (no error)"=w11, "M1M3SAL in"=w27) -> ()  [unwired: 8 in, 2 out]
  n162 = flat-sequence {
    tunnel: w11 -> [_]
    frame #0 {
      n163 = local write "Ready?"(TRUE ("Ready?")) -> ()
    }
  }
  n164 = while {
    shift-right: [w374] -> w26
    shift-left: w27 -> [w375]
    shift-right: [w372] -> w29
    shift-left: w11 -> [w373]
    stop <- w371 stop-if-true
    n165 = event shown="[4] \"TelemetryForceActuatorDataGo\": Value Change" {
      selector: _ -> [_ _ _ _ _ _ _ _ _ _ _]
      dyn-events: _ -> [_ _ _ _ _ _ _ _ _ _ _]
      timeout: _ -> [_ _ _ _ _ _ _ _ _ _ _]
      tunnel: w375 -> [w380 w385 w390 w394 w399 w434 w451 w456 w461 w488 w503]
      tunnel: [w379 w382 w389 w393 w396 w433 w448 w454 w459 w486 w503] -> w374
      tunnel: w373 -> [w378 w384 w388 w392 w398 w431 w450 w455 w460 w487 w502]
      tunnel: [w377 w383 w387 w391 w397 w432 w449 w453 w458 w485 w502] -> w372
      tunnel: [_ _ _ _ _ _ _ _ _ _ w504] -> w371
      event "TelemetryAirDataGo": Value Change {
        n166 = event-data() -> ()  [unwired: 1 in, 3 out]
        n167 = call-dynamic "putAirData.vi"("error in (no error)"=w378, "TelemetryAirData"=T5 {"Timestamp"=1.0, "CellAirPressure"=2.0, "HardpointAirPressure"=3.0}, "M1M3SAL in"=w380) -> ("error out"=w377:errorcluster, "M1M3SAL out"=w379:refnum<class "M1M3SAL.lvclass">)  [unwired: 7 in]
      }
      event "TelemetryIMSDataGo": Value Change {
        n168 = event-data() -> ()  [unwired: 1 in, 3 out]
        n169 = call-dynamic "putIMSData.vi"("error in (no error)"=w384, "TelemetryIMSData"=T6 {"Timestamp"=1.0, "XPosition"=2.0, "YPosition"=3.0, "ZPosition"=4.0, "XRotation"=5.0, "YRotation"=6.0, "ZRotation"=7.0}, "M1M3SAL in"=w385) -> ("error out"=w383:errorcluster, "M1M3SAL out"=w382:refnum<class "M1M3SAL.lvclass">)  [unwired: 7 in]
      }
      event "TelemetryDynamicDataGo": Value Change {
        n170 = event-data() -> ()  [unwired: 1 in, 3 out]
        n171 = call-dynamic "putDynamicData.vi"("error in (no error)"=w388, "TelemetryDynamicData"=T7 {"Timestamp"=1.0, "AzimuthVelocity"=2.0, "ElevationVelocity"=3.0, "AzimuthAcceleration"=4.0, "ElevationAcceleration"=5.0}, "M1M3SAL in"=w390) -> ("error out"=w387:errorcluster, "M1M3SAL out"=w389:refnum<class "M1M3SAL.lvclass">)  [unwired: 7 in]
      }
      event "TelemetryElevationDataGo": Value Change {
        n172 = event-data() -> ()  [unwired: 1 in, 3 out]
        n173 = call-dynamic "putElevationData.vi"("error in (no error)"=w392, "TelemetryElevationData"=T8 {"Timestamp"=1.0, "InclinometerElevation"=2.0, "MeasuredElevation"=3.0}, "M1M3SAL in"=w394) -> ("error out"=w391:errorcluster, "M1M3SAL out"=w393:refnum<class "M1M3SAL.lvclass">)  [unwired: 7 in]
      }
      event "TelemetryForceActuatorDataGo": Value Change {
        n174 = event-data() -> ()  [unwired: 1 in, 3 out]
        n175 = for {
          N: 156 -> [_]
          tunnel: [TRUE] -> w408 mode=indexing
          tunnel: [FALSE] -> w409 mode=indexing
          tunnel: [w427] -> w407 mode=indexing
          tunnel: [w425] -> w406 mode=indexing
          tunnel: [w420] -> w405 mode=indexing
          tunnel: [w419] -> w404 mode=indexing
          tunnel: [w418] -> w403 mode=indexing
          tunnel: [w417] -> w402 mode=indexing
          tunnel: [w413] -> w401 mode=indexing
          i -> [w416]
          n176 = To Unsigned Byte Integer(number=w416) -> (unsigned 8bit integer=w415:u8)
          n177 = Add(x=3.0, y=w416) -> (x+y=w427:dbl)
          n178 = Add(x=4.0, y=w416) -> (x+y=w425:dbl)
          n179 = Add(x=sgl 7.0, y=w416) -> (x+y=w418:sgl)
          n180 = Add(x=5.0, y=w416) -> (x+y=w420:dbl)
          n181 = Add(x=sgl 6.0, y=w416) -> (x+y=w419:sgl)
          n182 = Add(x=sgl 8.0, y=w416) -> (x+y=w417:sgl)
          n183 = Add(x=u8 11, y=w415) -> (x+y=w413:u8)
        }
        n184 = Bundle By Name(cluster=T9 {"Timestamp"=0.0, "SlewFlagCommanded"=[], "XSetpointCommanded"=[], "YSetpointCommanded"=[], "ZSetpointCommanded"=[], "XForce"=[], "YForce"=[], "ZForce"=[], "ILCFault"=[], "DCAFault"=[], "BroadcastCounter"=[]} ("TelemetryForceActuatorData"), "Timestamp"=T3 1.0, "SlewFlagCommanded"=w408, "XSetpointCommanded"=w407, "YSetpointCommanded"=w406, "ZSetpointCommanded"=w405, "XForce"=w404, "YForce"=w403, "ZForce"=w402, "ILCFault"=w409, "DCAFault"=w408, "BroadcastCounter"=w401) -> (w400:T9)
        n185 = call-dynamic "putForceActuatorData.vi"("error in (no error)"=w398, "TelemetryForceActuatorData"=w400, "M1M3SAL in"=w399) -> ("error out"=w397:errorcluster, "M1M3SAL out"=w396:refnum<class "M1M3SAL.lvclass">)  [unwired: 7 in]
      }
      event "TelemetryForceActuatorStatusGo": Value Change {
        n186 = event-data() -> ()  [unwired: 1 in, 3 out]
        n187 = for {
          N: 156 -> [_]
          tunnel: [w444] -> w438 mode=indexing
          tunnel: [TRUE] -> w437 mode=indexing
          tunnel: [FALSE] -> w436 mode=indexing
          i -> [w447]
          n188 = To Unsigned Byte Integer(number=w447) -> (unsigned 8bit integer=w446:u8)
          n189 = Add(x=u8 2, y=w446) -> (x+y=w444:u8)
        }
        n190 = Bundle By Name(cluster=T10 {"Timestamp"=0.0, "Mode"=[], "MajorFault"=[], "MinorFault"=[], "FaultOverridden"=[], "DCAFault"=[], "WatchdogReset"=[], "BrownoutDetected"=[], "EventTrapReset"=[], "MotorPowerFault"=[], "SSRPowerFault"=[], "AUXPowerFault"=[], "SMCPowerFault"=[], "DCAOutputsEnabled"=[], "DCAPowerFault"=[], "DCAAmplifierAFault"=[], "DCAAmplifierBFault"=[], "DCAEventTrapReset"=[]} ("TelemetryForceActuatorStatus"), "Timestamp"=T3 1.0, "Mode"=w438, "MajorFault"=w437, "MinorFault"=w436, "FaultOverridden"=w437, "DCAFault"=w436, "WatchdogReset"=w437, "BrownoutDetected"=w436, "EventTrapReset"=w437, "MotorPowerFault"=w436, "SSRPowerFault"=w437, "AUXPowerFault"=w436, "SMCPowerFault"=w437, "DCAOutputsEnabled"=w436, "DCAPowerFault"=w437, "DCAAmplifierAFault"=w436, "DCAAmplifierBFault"=w437, "DCAEventTrapReset"=w436) -> (w435:T10)
        n191 = call-dynamic "putForceActuatorStatus.vi"("error in (no error)"=w431, "TelemetryForceActuatorStatus"=w435, "M1M3SAL in"=w434) -> ("error out"=w432:errorcluster, "M1M3SAL out"=w433:refnum<class "M1M3SAL.lvclass">)  [unwired: 7 in]
      }
      event "TelemetryFPGADataGo": Value Change {
        n192 = event-data() -> ()  [unwired: 1 in, 6 out]
        n193 = call-dynamic "putFPGAData.vi"("error in (no error)"=w450, "TelemetryFPGAData"=T11 {"Timestamp"=1.0, "ModbusSubnetATxInternalFIFOOverflow"=TRUE, "ModbusSubnetAInvalidInstruction"=FALSE, "ModbusSubnetAWaitForRxFrameTimeout"=TRUE, "ModbusSubnetAStartBitError"=FALSE, "ModbusSubnetAStopBitError"=TRUE, "ModbusSubnetARxDataFIFOOverflow"=FALSE, "ModbusSubnetATxByteCount"=8, "ModbusSubnetATxFrameCount"=9, "ModbusSubnetARxByteCount"=10, "ModbusSubnetARxFrameCount"=11, "ModbusSubnetBTxInternalFIFOOverflow"=TRUE, "ModbusSubnetBInvalidInstruction"=FALSE, "ModbusSubnetBWaitForRxFrameTimeout"=TRUE, "ModbusSubnetBStartBitError"=FALSE, "ModbusSubnetBStopBitError"=TRUE, "ModbusSubnetBRxDataFIFOOverflow"=FALSE, "ModbusSubnetBTxByteCount"=18, "ModbusSubnetBTxFrameCount"=19, "ModbusSubnetBRxByteCount"=20, "ModbusSubnetBRxFrameCount"=21, "ModbusSubnetCTxInternalFIFOOverflow"=TRUE, "ModbusSubnetCInvalidInstruction"=FALSE, "ModbusSubnetCWaitForRxFrameTimeout"=TRUE, "ModbusSubnetCStartBitError"=FALSE, "ModbusSubnetCStopBitError"=TRUE, "ModbusSubnetCRxDataFIFOOverflow"=FALSE, "ModbusSubnetCTxByteCount"=28, "ModbusSubnetCTxFrameCount"=29, "ModbusSubnetCRxByteCount"=30, "ModbusSubnetCRxFrameCount"=31, "ModbusSubnetDTxInternalFIFOOverflow"=TRUE, "ModbusSubnetDInvalidInstruction"=FALSE, "ModbusSubnetDWaitForRxFrameTimeout"=TRUE, "ModbusSubnetDStartBitError"=FALSE, "ModbusSubnetDStopBitError"=TRUE, "ModbusSubnetDRxDataFIFOOverflow"=FALSE, "ModbusSubnetDTxByteCount"=38, "ModbusSubnetDTxFrameCount"=39, "ModbusSubnetDRxByteCount"=40, "ModbusSubnetDRxFrameCount"=41, "ModbusSubnetETxInternalFIFOOverflow"=TRUE, "ModbusSubnetEInvalidInstruction"=FALSE, "ModbusSubnetEWaitForRxFrameTimeout"=TRUE, "ModbusSubnetEStartBitError"=FALSE, "ModbusSubnetEStopBitError"=TRUE, "ModbusSubnetERxDataFIFOOverflow"=FALSE, "ModbusSubnetETxByteCount"=48, "ModbusSubnetETxFrameCount"=49, "ModbusSubnetERxByteCount"=50, "ModbusSubnetERxFrameCount"=51, "FPGATimestamp"=52.0}, "M1M3SAL in"=w451) -> ("error out"=w449:errorcluster, "M1M3SAL out"=w448:refnum<class "M1M3SAL.lvclass">)  [unwired: 7 in]
      }
      event "TelemetryMirrorForceDataGo": Value Change {
        n194 = event-data() -> ()  [unwired: 1 in, 6 out]
        n195 = call-dynamic "putMirrorForceData.vi"("error in (no error)"=w455, "TelemetryMirrorForceData"=T12 {"Timestamp"=1.0, "Fx"=2.0, "Fy"=3.0, "Fz"=4.0, "Mx"=5.0, "My"=6.0, "Mz"=7.0}, "M1M3SAL in"=w456) -> ("error out"=w453:errorcluster, "M1M3SAL out"=w454:refnum<class "M1M3SAL.lvclass">)  [unwired: 7 in]
      }
      event "TelemetryHardpointData": Value Change {
        n196 = event-data() -> ()  [unwired: 1 in, 6 out]
        n197 = for {
          N: 6 -> [_]
          tunnel: [w482] -> w468 mode=indexing
          tunnel: [w480] -> w467 mode=indexing
          tunnel: [w478] -> w466 mode=indexing
          tunnel: [TRUE] -> w465 mode=indexing
          tunnel: [FALSE] -> w464 mode=indexing
          tunnel: [w472] -> w463 mode=indexing
          i -> [w475]
          n198 = To Word Integer(number=w475) -> (16bit integer=w484:i16)
          n199 = To Unsigned Byte Integer(number=w475) -> (unsigned 8bit integer=w474:u8)
          n200 = Add(x=sgl 3.0, y=w475) -> (x+y=w480:sgl)
          n201 = Add(x=4, y=w475) -> (x+y=w478:i32)
          n202 = Add(x=i16 2, y=w484) -> (x+y=w482:i16)
          n203 = Add(x=u8 8, y=w474) -> (x+y=w472:u8)
        }
        n204 = Bundle By Name(cluster=T13 {"Timestamp"=0.0, "StepsCommanded"=[], "Force"=[], "Encoder"=[], "ILCFault"=[], "CWLimitOperated"=[], "CCWLimitOperated"=[], "BroadcastCounter"=[]} ("TelemetryHardpointData"), "Timestamp"=T3 1.0, "StepsCommanded"=w468, "Force"=w467, "Encoder"=w466, "ILCFault"=w465, "CWLimitOperated"=w464, "CCWLimitOperated"=w465, "BroadcastCounter"=w463) -> (w462:T13)
        n205 = call-dynamic "putHardpointData.vi"("error in (no error)"=w460, "TelemetryHardpointData"=w462, "M1M3SAL in"=w461) -> ("error out"=w458:errorcluster, "M1M3SAL out"=w459:refnum<class "M1M3SAL.lvclass">)  [unwired: 7 in]
      }
      event "TelemetryHardpointStatus": Value Change {
        n206 = event-data() -> ()  [unwired: 1 in, 6 out]
        n207 = for {
          N: 6 -> [_]
          tunnel: [w498] -> w492 mode=indexing
          tunnel: [TRUE] -> w491 mode=indexing
          tunnel: [FALSE] -> w490 mode=indexing
          i -> [w501]
          n208 = To Unsigned Byte Integer(number=w501) -> (unsigned 8bit integer=w500:u8)
          n209 = Add(x=u8 2, y=w500) -> (x+y=w498:u8)
        }
        n210 = Bundle By Name(cluster=T14 {"Timestamp"=0.0, "Mode"=[], "MajorFault"=[], "MinorFault"=[], "FaultOverridden"=[], "WatchdogReset"=[], "BrownoutDetected"=[], "EventTrapReset"=[], "MotorPowerFault"=[], "SSRPowerFault"=[], "AUXPowerFault"=[], "SMCPowerFault"=[]} ("TelemetryHardpointStatus"), "Timestamp"=T3 1.0, "Mode"=w492, "MajorFault"=w491, "MinorFault"=w490, "FaultOverridden"=w491, "WatchdogReset"=w490, "BrownoutDetected"=w491, "EventTrapReset"=w490, "MotorPowerFault"=w491, "SSRPowerFault"=w490, "AUXPowerFault"=w491, "SMCPowerFault"=w490) -> (w489:T14)
        n211 = call-dynamic "putHardpointStatus.vi"("error in (no error)"=w487, "TelemetryHardpointStatus"=w489, "M1M3SAL in"=w488) -> ("error out"=w485:errorcluster, "M1M3SAL out"=w486:refnum<class "M1M3SAL.lvclass">)  [unwired: 7 in]
      }
      event "Stop": Value Change {
        n212 = event-data() -> ()  [unwired: 1 in, 3 out]
        n213 = local read "Stop"() -> (w504:bool)
      }
    }
  }
  n214 = call "generateInternalShutdown.vi"("error in (no error)"=w29, "ShutdownEvent"=T1 {"Shutdown"=TRUE}, "UserEvents in"=w22) -> ("error out"=w25:errorcluster, "UserEvents out"=w24:refnum<class "UserEvents.lvclass">)  [unwired: 7 in]
  n215 = call-dynamic "stopService.vi"("error in (no error)"=w25, "M1M3SAL in"=w26) -> ("error out"=w23:errorcluster)  [unwired: 8 in, 1 out]
  n216 = call "destroyUserEvents.vi"("error in (no error)"=w23, "UserEvents in"=w24) -> ()  [unwired: 8 in, 2 out]
  "Ready?" <- FALSE ("Ready?")
